vi "Quadrotor MPU6050.vi"() -> ()   [LabVIEW 2013]
uses:
  <vilib>/Platform/TimedLoop/XDataNode/timing_clust.ctl
  <vilib>/Platform/TimedLoop/XDataNode/nitl_modes.ctl
  <vilib>/Platform/TimedLoop/XDataNode/wakeup.ctl
  <vilib>/FPGAPlugInAG/myRIO-1900/niLvFpga_Open_myRIO-1900.vi
  <vilib>/rvi/interface/common/dynamic/niFpgaDynamicAddResources.vi
  <vilib>/myRIO/Common/Instrument Driver Framework/Utilities/vis/FPGA Ref Manager.vi
  <vilib>/Utility/error.llb/Error Cluster From Error Code.vi
  <vilib>/FPGAPlugInAG/Dynamic/niLvFpga_Close_Dynamic.vi
  <vilib>/rvi/interface/nirviOpenFPGA/nirviOpenFPGA.xnode
  FPGA Bitfiles/MyThirdNImyRIOPr_FPGATarget_myRIO-1900Quadro_CJ6JRY0Vo8Q.lvbitx
  <vilib>/Platform/TimedLoop/XDataNode/XDataNode.xnode
  <vilib>/rvi/interface/nirviCloseFPGA/nirviCloseFPGA.xnode
  <vilib>/myRIO/Instrument Drivers/Utilities/Utilities.lvlib
  <vilib>/Platform/TimedLoop/XDataNode/XDNodeRunTimeDep.lvlib
panel:
  out "GYR":cluster{"GYR_X":i16, "GYR_Y":i16, "GYR_Z":i16}(graph)
  out "ACC":cluster{"ACC_X":i16, "ACC_Y":i16, "ACC_Z":i16}(graph)
  out "TEMP":i16
  out "error out":errorcluster
  in  "Stop Button":bool
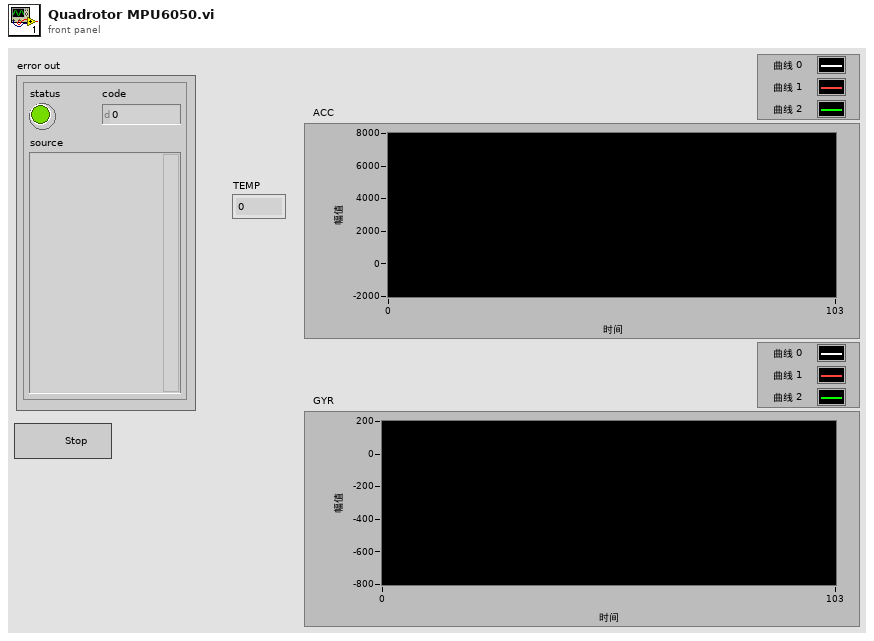
[diagram p1: front panel]
types:
  T1 = typedef "XDNodeRunTimeDep.lvlib/timing_clust.ctl" = cluster{"Expected End [f-1]":u64, "Actual End [f-1]":u64, "Finished Late? [f-1]":bool, "Expected End [i-1]":u64, "Actual End [i-1]":u64, "Finished Late? [i-1]":bool, "Expected Start [i]":u64, "Actual Start [i]":u64, "Expected Start [f]":u64, "Actual Start [f]":u64, "Source Name":string, "Structure Name":string, "Period":i64, "Deadline":i64, "Offset":i64, "Start":i64, "Priority":i32, "Timeout":i32, "Mode":T2, "Wakeup Reason":T3, "Error":errorcluster, "Source Type":string, "Secondary Source Type":string, "Global End Time":u64, "Global Start Time":u64, "Frame Duration":u64, "Iteration Duration":u64, "Assigned CPU":i32, "I/O Scan Engine Mode":u32}
  T2 = typedef "XDNodeRunTimeDep.lvlib/nitl_modes.ctl" = enum32{"No Change", "Process missed periods, maintain original phase", "Discard missed periods, maintain original phase", "Process missed periods, ignore original phase", "Discard missed periods, ignore original phase"}
  T3 = typedef "XDNodeRunTimeDep.lvlib/wakeup.ctl" = enum32{"Normal", "Aborted", "Asynchronous wakeup", "Timing source error", "Timed loop error", "Timeout"}
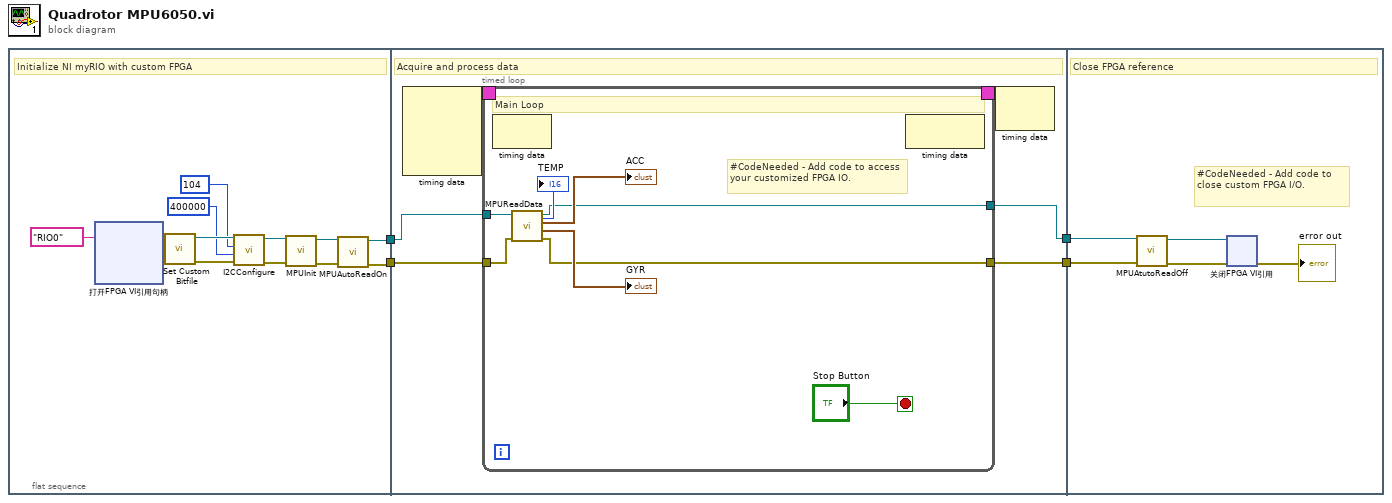
[diagram p0: block diagram]
diagram:
  n1 = flat-sequence {
    tunnel: [w5] -> w4
    tunnel: [w8] -> w3
    tunnel: w4 -> [w21]
    tunnel: [w18] -> w2
    tunnel: w3 -> [w20]
    tunnel: [w19] -> w1
    tunnel: w2 -> [w39]
    tunnel: w1 -> [w37]
    frame #0 {
      # "Initialize NI myRIO with custom FPGA"
      n2 = xnode "打开FPGA VI引用句柄"("资源名称"=tag "RIO0" ("resource name")) -> ("FPGA VI引用输出"=w15:refnum<k20>, "错误输出"=w16:errorcluster)  [unwired: 1 in]
      n3 = call <vilib>:"Set Custom Bitfile.vi"("error in (no error)"=w16, "Customized FPGA Reference in"=w15) -> ("error out"=w13:errorcluster, "Customized FPGA Reference out"=w14:refnum<k20>)  [unwired: 8 in]
      n4 = call "I2CConfigure.vi"("error in (no error)"=w13, "Clock Rate"=u32 400000, "IICSlaveAddress"=u16 104, "FPGA VI引用输入"=w14) -> ("error out"=w10:errorcluster, "FPGA VI引用输出"=w7:refnum<k20>)  [unwired: 6 in]
      n5 = call "MPUInit.vi"("ErrorIn(no error)"=w10, "FPGA VI引用输入"=w7) -> ("ErrorOut"=w9:errorcluster, "FPGA VI引用输出"=w6:refnum<k20>)  [unwired: 8 in]
      n6 = call "MPUAutoReadOn.vi"("ErrorIn(no error)"=w9, "FPGA VI引用输入"=w6) -> ("ErrorOut"=w8:errorcluster, "FPGA VI引用输出"=w5:refnum<k20>)  [unwired: 8 in]
    }
    frame #1 {
      # "Acquire and process data"
      n7 = node-c288() -> (w23:T1)  [unwired: 4 in]
      n8 = timed-loop {
        timing: w23 -> [_]
        timing-out: [_] -> w22
        tunnel: w21 -> [w27]
        tunnel: w20 -> [w26]
        tunnel: [w25] -> w19
        tunnel: [w24] -> w18
        stop <- "Stop Button" stop-if-true
        # "#CodeNeeded - Add code to access your customized FPGA IO."
        # "Main Loop"
        n9 = node-c288() -> ()  [unwired: 1 in, 1 out]
        n10 = call "MPUReadData.vi"("ErrorIn"=w26, "FPGA VI引用输入"=w27) -> ("ErrorOut"=w24:errorcluster, "GYR"=→"GYR":cluster{"GYR_X":i16, "GYR_Y":i16, "GYR_Z":i16}, "ACC"=→"ACC":cluster{"ACC_X":i16, "ACC_Y":i16, "ACC_Z":i16}, "FPGA VI引用输出"=w25:refnum<k20>, "TEMP"=→"TEMP":i16)  [unwired: 5 in]
        n11 = node-c288() -> ()  [unwired: 1 in, 1 out]
      }
      n12 = node-c288(w22) -> ()  [unwired: 1 out]
    }
    frame #2 {
      # "#CodeNeeded - Add code to close custom FPGA I/O."
      # "Close FPGA reference"
      n13 = call "MPUAtutoReadOff.vi"("ErrorIn(no error)"=w39, "FPGA VI引用输入"=w37) -> ("ErrorOut"=w38:errorcluster, "FPGA VI引用输出"=w36:refnum<k20>)  [unwired: 8 in]
      n14 = xnode "关闭FPGA VI引用"("FPGA VI引用输入"=w36, "错误输入"=w38) -> ("错误输出"=→"error out":errorcluster)
    }
  }
